vi "Inv F Distribution.vi"(2 "m":i32=1 format="%0.0f", 3 "n":i32=1 format="%0.0f", 4 "probability":dbl format="%0.4f") -> (0 "error":i32, 1 "x":dbl format="%0.4f")   [LabVIEW 2014, in "NI_AALPro.lvlib"]
doc: "LabVIEW no longer supports this VI. Use the Continuous Inverse CDF VI (F instance) instead. Computes the value of <B>x</B> given the <B>probability</B> value p of an F-distributed random variable F with <B>n</B> and <B>m</B> degrees of freedom. The Inv F Distribution VI computes the value of <B>x</B> such that the following condition is satisfied: p = Prob{F[<B>n</B>, <B>m</B>] < <B>x</B>}, where F is F-distributed, p is the <B>probability</B>, <B>n</B> specifies the first degree of freedom, <B>m</B> specifies the second degree of freedom, and <B>x</B> is the value."
uses:
  NI_AALPro.lvlib
  lvanlys.dll
panel:
  # "Inverse F Distribution"
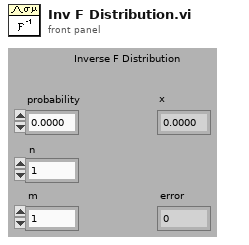
[diagram p1: front panel]
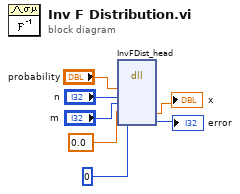
[diagram p0: block diagram]
diagram:
  n1 = dll-call lib="C:/Program Files (x86)/National Instruments/LabVIEW 2014/resource/lvanlys.*" fn="InvFDist_head"("probability"="probability", "n"="n", "m"="m", 0.0, 0) -> (→"x":dbl, →"error":i32)  [unwired: 7 in, 2 out]
